vi "UART Configure Stop Bits.vi"(0 "UART Driver in":refnum<class "UART Driver.lvclass">, 1 "Port Number":u8, 5 "Stop Bits":T1, 11 "error in":errorcluster) -> (4 "UART Driver out":refnum<class "UART Driver.lvclass">, 6 "Receive Data":string, 15 "error out":errorcluster)   [LabVIEW 2012, in "UART_Host_Driver.lvlib" / "UART Driver.lvclass"]
doc: "Configure the Stop Bit/s.\n\nMust call UART Initialize.vi, prior to calling UART Configure Stop Bits.vi.\n\nNote: Port Number 255 means to transmit to all of the ports configured in the UART Initialize.vi."
uses:
  UART Driver.lvclass
  FPGA/UART/StopBits.ctl
  FPGA/UART/UART_Command.ctl
  UART Driver.lvclass/UART Driver.ctl
  Typedefs/FPGA VI Reference.ctl
  <vilib>/Utility/error.llb/Error Cluster From Error Code.vi
  <vilib>/rvi/errors/niLvFpgaAdjustHostInterfaceError.vi
  <vilib>/rvi/interface/nirviMethod/nirviMethod.xnode
  UART_Host_Driver.lvlib
  <vilib>/FPGAPlugInAG/Dynamic/niLvFpga_WriteFifo_Dynamic.vi
  <vilib>/rvi/errors/niLvFpgaMergeErrorWithErrorCode.vi
  FPGA/UART/UART_Firmware.lvlib
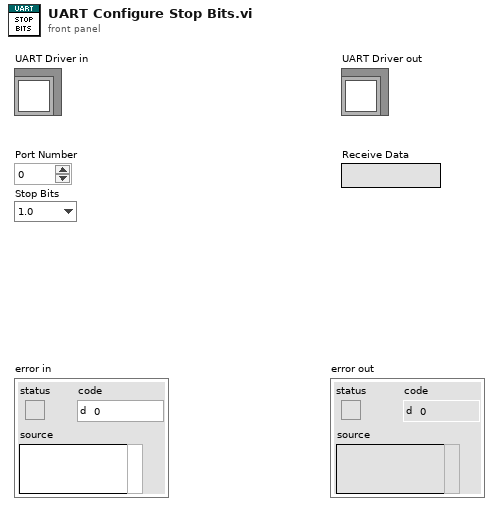
[diagram p1: front panel]
types:
  T1 = typedef "UART_Firmware.lvlib/StopBits.ctl" = enum8{"1.0", "1.5", "2.0"}
  T2 = typedef "UART_Firmware.lvlib/UART_Command.ctl" = enum8{"None", "Tx", "SetBaud_High", "SetBaud_Low", "SetCharLength", "SetParity", "SetStopBits", "SetSpacing_High", "SetSpacing_Low"}
  T3 = typedef "UART_Host_Driver.lvlib/FPGA VI Reference.ctl" = refnum<k20>
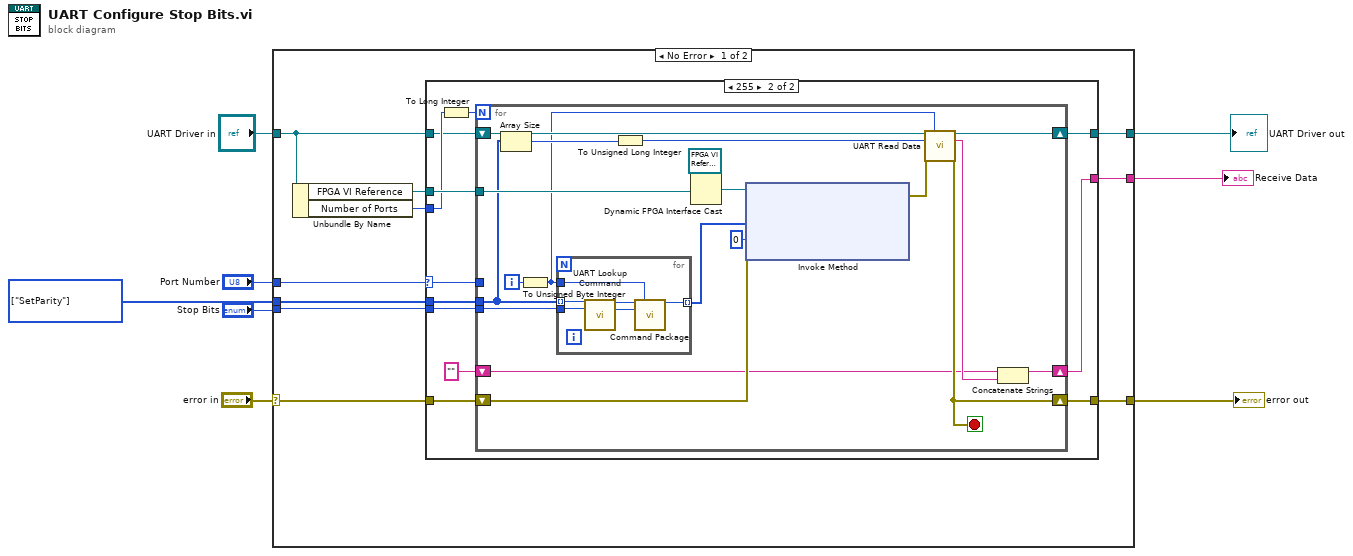
[diagram p0: block diagram]
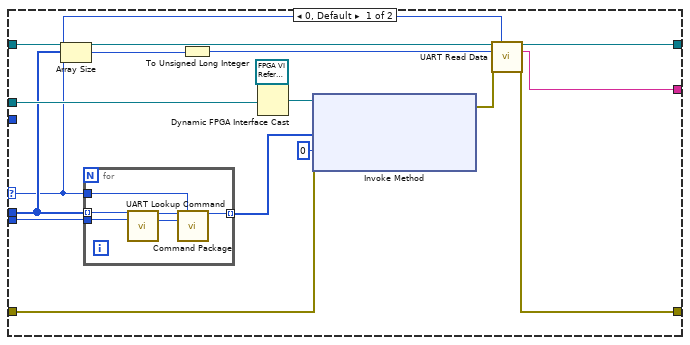
[diagram p2: hidden frame]
diagram:
  w2 = T2[] [enum."SetParity"] items=["None", "Tx", "SetBaud_High", "SetBaud_Low", "SetCharLength", "SetParity", "SetStopBits", "SetSpacing_High", "SetSpacing_Low"] ("Input Parameters")
  n1 = case shown="No Error" "error in" {
    selector: "error in" -> [w16 w79]
    tunnel: [w13 w79] -> w7
    tunnel: [w14 w78] -> w5
    tunnel: "UART Driver in" -> [w15 w78]
    tunnel: "Stop Bits" -> [w18 _]
    tunnel: w2 -> [w11 _]
    tunnel: [w12 _] -> w4
    tunnel: "Port Number" -> [w10 _]
    frame No Error {
      n2 = Unbundle By Name(w15) -> ("FPGA VI Reference"=w17:refnum<k20>, "Number of Ports"=w9:u8)
      n3 = case shown="255" w10 {
        selector: w10 -> [w19 w46]
        tunnel: w18 -> [w34 w52]
        tunnel: w17 -> [w31 w51]
        tunnel: w16 -> [w28 w50]
        tunnel: w15 -> [w27 w43]
        tunnel: [w26 w49] -> w14
        tunnel: [w24 w48] -> w13
        tunnel: [w23 w41] -> w12
        tunnel: w11 -> [w22 w47]
        tunnel: w9 -> [_ w45]
        frame 0, Default {
          n4 = Array Size(array=w22) -> (size(s)=w21:i32)
          n5 = for {
            tunnel: w34 -> [w40]
            tunnel: [w37] -> w32 mode=indexing
            tunnel: w22 -> [w36] mode=indexing
            tunnel: w19 -> [w35]
            n6 = call "UART Lookup Command.vi"("UART_Command in"=w36, "Baud"=w40) -> ("UART_Command out"=w39:T2, "Numeric"=w38:u16)  [unwired: 12 in]
            n7 = call "Command Package.vi"("UART_Command"=w39, "Channel Number"=w35, "Cmd_data"=w38) -> ("Cmd_package"=w37:u32)  [unwired: 12 in]
          }
          n8 = To Unsigned Long Integer(number=w21) -> (unsigned 32bit integer=w20:u32)
          n9 = Dynamic FPGA Interface Cast(Session In=T3 refnum ("FPGA VI Reference"), Type=w31) -> (Session Out=w30:T3)
          n10 = xnode "Invoke Method"("FPGA VI Reference In"=w30, "error in"=w28, "Data"=w32, "Timeout (ms)"=0) -> ("error out"=w25:errorcluster)  [unwired: 2 out]
          n11 = call-dynamic "UART Read Data.vi"("UART Driver in"=w27, "Port Number"=w19, "Rx byte count"=w20, "error in"=w25) -> ("UART Driver out"=w26:refnum<class "UART Driver.lvclass">, "Receive Data"=w23:string, "error out"=w24:errorcluster)  [unwired: 9 in]
        }
        frame 255 {
          n12 = To Long Integer(number=w45) -> (32bit integer=w44:i32)
          n13 = for {
            N: w44 -> [_]
            tunnel: w52 -> [w71]
            tunnel: w51 -> [w68]
            tunnel: w47 -> [w62]
            tunnel: w46 -> [_]
            shift-right: [w64] -> w49
            shift-left: w43 -> [w59]
            shift-right: [w58] -> w48
            shift-left: w50 -> [w65]
            shift-right: [w55] -> w41
            shift-left: "" -> [w56]
            i -> [w54]
            stop <- w58 stop-if-true
            n14 = Array Size(array=w62) -> (size(s)=w61:i32)
            n15 = To Unsigned Byte Integer(number=w54) -> (unsigned 8bit integer=w53:u8)
            n16 = for {
              tunnel: w71 -> [w77]
              tunnel: [w74] -> w69 mode=indexing
              tunnel: w62 -> [w73] mode=indexing
              tunnel: w53 -> [w72]
              n17 = call "UART Lookup Command.vi"("UART_Command in"=w73, "Baud"=w77) -> ("UART_Command out"=w76:T2, "Numeric"=w75:u16)  [unwired: 12 in]
              n18 = call "Command Package.vi"("UART_Command"=w76, "Channel Number"=w72, "Cmd_data"=w75) -> ("Cmd_package"=w74:u32)  [unwired: 12 in]
            }
            n19 = To Unsigned Long Integer(number=w61) -> (unsigned 32bit integer=w60:u32)
            n20 = Dynamic FPGA Interface Cast(Session In=T3 refnum ("FPGA VI Reference"), Type=w68) -> (Session Out=w67:T3)
            n21 = xnode "Invoke Method"("FPGA VI Reference In"=w67, "error in"=w65, "Data"=w69, "Timeout (ms)"=0) -> ("error out"=w63:errorcluster)  [unwired: 2 out]
            n22 = call-dynamic "UART Read Data.vi"("UART Driver in"=w59, "Port Number"=w53, "Rx byte count"=w60, "error in"=w63) -> ("UART Driver out"=w64:refnum<class "UART Driver.lvclass">, "Receive Data"=w57:string, "error out"=w58:errorcluster)  [unwired: 9 in]
            n23 = Concatenate Strings(w56, w57) -> (w55:string)
          }
        }
      }
    }
    frame Error {
    }
  }
  "error out" <- w7
  "UART Driver out" <- w5
  "Receive Data" <- w4
